vi "write TBM configuration.vi"(8 "error in":errorcluster, 10 "TBM configuration in":refnum<class "TBM configuration.lvclass">, 11 "EthernetIP editor node in":refnum<class "EthernetIP editor node.lvclass">) -> (0 "error out":errorcluster, 3 "EthernetIP editor node out":refnum<class "EthernetIP editor node.lvclass">)   [LabVIEW 2013, in "EthernetIP editor node.lvclass"]
uses:
  EthernetIP editor node.lvclass
  <vilib>/NI/Tag Bus Module Framework/root configuration/TBM configuration.lvclass
  <vilib>/NI/TBM Modules/Ethernet IP/configuration/EthernetIP configuration.lvclass
  EthernetIP editor node.lvclass/EthernetIP editor node.ctl
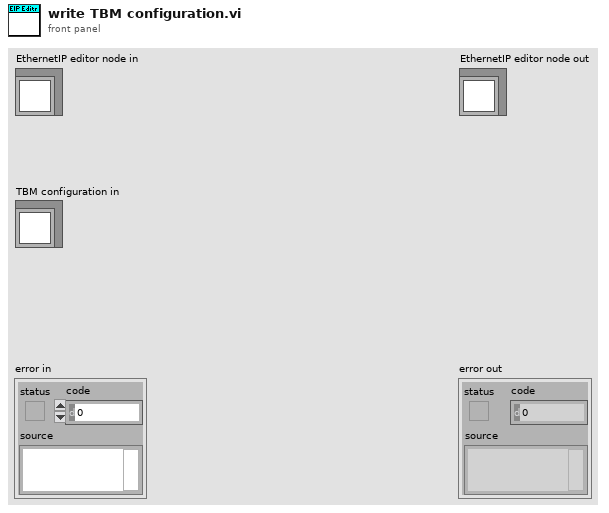
[diagram p1: front panel]
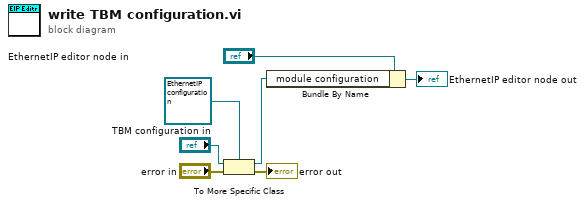
[diagram p0: block diagram]
diagram:
  n1 = To More Specific Class(target class=refnum<class "EthernetIP configuration.lvclass"> refnum ("module configuration"), reference="TBM configuration in", error in="error in") -> (specific class reference=w1:refnum<class "EthernetIP configuration.lvclass">, error out=→"error out":errorcluster)
  n2 = Bundle By Name(cluster="EthernetIP editor node in", "module configuration"=w1) -> (→"EthernetIP editor node out":refnum<class "EthernetIP editor node.lvclass">)
